vi "SaveStoppanniFile.vi"(8 "Last Path":path=path "/Users/crogers/Desktop/Curtin2/Data/ScratchPad/Raw/Medium Hit 000_000_000.wav", 9 "Coherence in":cluster{"x0":dbl, "df":dbl, dbl[]}, 10 "Inst:Test Name":string, 11 "Complex FRF":cluster{"t0":dbl, "dt":dbl, "Y":cdb[]}) -> (0 "trf file":path)   [LabVIEW 2022 SP3]
panel:
  out "error out":errorcluster
  out "Header Info":T1
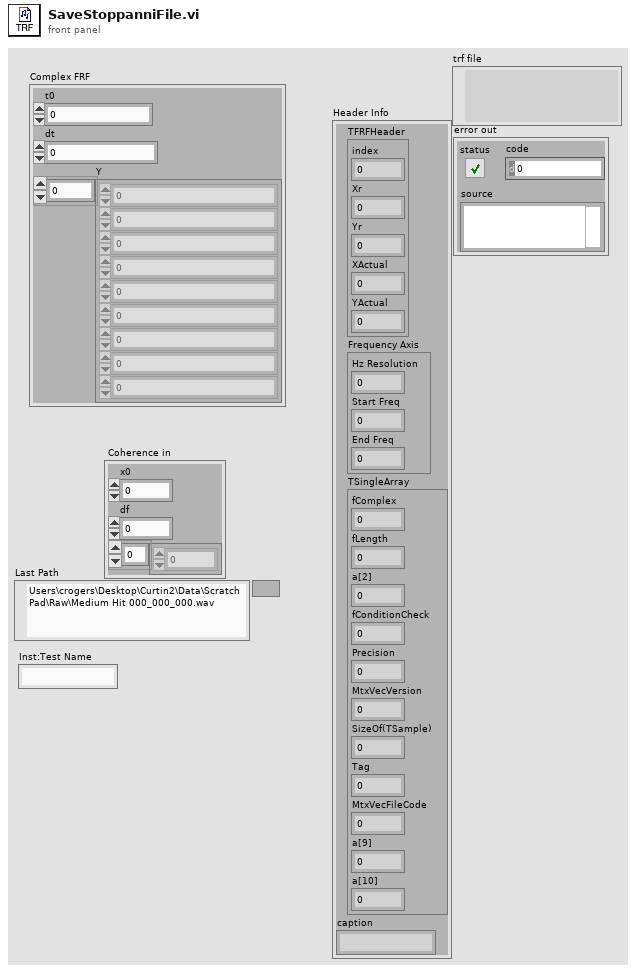
[diagram p1: front panel]
types:
  T1 = cluster{"TFRFHeader":cluster{"index":u32, "Xr":dbl, "Yr":dbl, "XActual":dbl, "YActual":dbl}, "Frequency Axis":cluster{"Hz Resolution":dbl, "Start Freq":dbl, "End Freq":dbl}, "TSingleArray":cluster{"fComplex":u32, "fLength":dbl, "a[2]":dbl, "fConditionCheck":dbl, "Precision":dbl, "MtxVecVersion":dbl, "SizeOf(TSample)":dbl, "Tag":dbl, "MtxVecFileCode":dbl, "a[9]":dbl, "a[10]":dbl}, "caption":string}
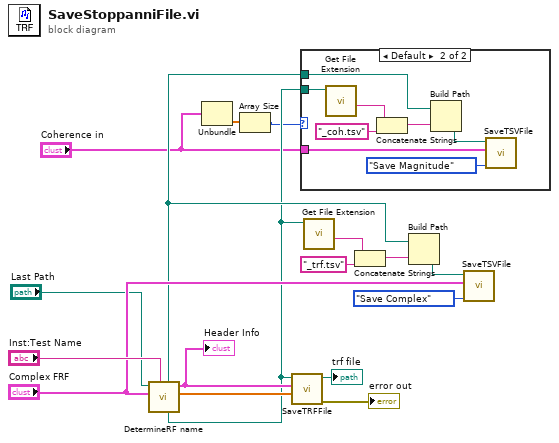
[diagram p0: block diagram]
diagram:
  n1 = call "DetermineRF name.vi"("Inst:Test Name"="Inst:Test Name", "Complex FRF"="Complex FRF", "Last Path"="Last Path") -> ("Y"=w16:cdb[], "Header Info"=w17:T1, "trf file"=w4:path, "Path to csv Folder"=w5:path)  [unwired: 5 in]
  "Header Info" <- w17
  n2 = Unbundle("Coherence in") -> (w2:dbl[])  [unwired: 2 out]
  n3 = Array Size(array=w2) -> (size(s)=w1:i32)
  n4 = call "SaveTRFFile.vi"("Y"=w16, "Header Info"=w17, "trf file in"=w4) -> ("error out"=→"error out":errorcluster, "trf file out"=→"trf file":path)  [unwired: 7 in]
  n5 = case shown="Default" w1 {
    tunnel: w5 -> [_ w20]
    tunnel: w4 -> [_ w19]
    tunnel: "Coherence in" -> [_ w18]
    frame 0 {
    }
    frame Default {
      n6 = call <vilib>:"Get File Extension.vi"("file"=w19) -> ("filename without extension"=w21:string)  [unwired: 6 in, 4 out]
      n7 = Concatenate Strings(w21, "_coh.tsv" ("string")) -> (w23:string)
      n8 = Build Path(base path=w20, name or relative path=w23) -> (appended path=w24:path)
      n9 = call "SaveTSVFile.vi"("Task"=enum16{"Save Magnitude", "Save Complex"}."Save Magnitude", "FRF"=w18, "Path"=w24) -> ()  [unwired: 8 in, 1 out]
    }
  }
  n10 = call <vilib>:"Get File Extension.vi"("file"=w4) -> ("filename without extension"=w14:string)  [unwired: 6 in, 4 out]
  n11 = Concatenate Strings(w14, "_trf.tsv" ("string")) -> (w12:string)
  n12 = Build Path(base path=w5, name or relative path=w12) -> (appended path=w11:path)
  n13 = call "SaveTSVFile.vi"("Task"=enum16{"Save Magnitude", "Save Complex"}."Save Complex", "FRF"="Complex FRF", "Path"=w11) -> ()  [unwired: 8 in, 1 out]
